vi "nxtxbool.vi"(11 "NXT In":T1={"Hardware"="NXT", "Flattened String"=""}) -> (3 "Chain Out":bool)   [LabVIEW 2010, in "LASA Beta.lvrbt"]
uses:
  LASA Beta.lvrbt
  <vilib>/NXT/Subs/LVHSConnector.ctl
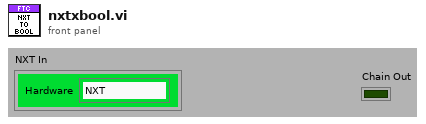
[diagram p1: front panel]
types:
  T1 = typedef "LVHSConnector.ctl" = cluster{"Hardware":string, "Flattened String":string}
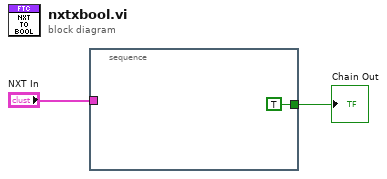
[diagram p0: block diagram]
diagram:
  n1 = stacked-sequence {
    tunnel: "NXT In" -> [_]
    tunnel: [TRUE] -> w1
    frame #0 {
    }
  }
  "Chain Out" <- w1
